vi "CloseDigitizerHandle.vi"() -> ()   [LabVIEW 2020]
panel:
  out "error out":errorcluster
  in  "instrument handle":refnum<k15>
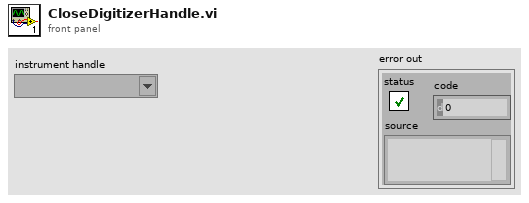
[diagram p1: front panel]
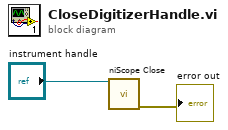
[diagram p0: block diagram]
diagram:
  n1 = call <instrlib>:"niScope Close.vi"("instrument handle"="instrument handle") -> ("error out"=→"error out":errorcluster)  [unwired: 14 in]
